vi "Kalman filter_STL.vi"(6 "Previous predicted pixel value":u16, 7 "Kalman gain":fxp<+,16,1>=0.1015625, 8 "Frame number":i32, 9 "Filter gain":fxp<+,16,0>=0.8000030517578125, 10 "Pixel value":u16, 11 "Input valid":bool=TRUE) -> (0 "Kalman filter result":u16, 1 "loop count":i32, 3 "output valid":bool)   [LabVIEW 2015]
uses:
  <vilib>/Platform/TimedLoop/XDataNode/timing_clust.ctl
  <vilib>/Platform/TimedLoop/XDataNode/nitl_modes.ctl
  <vilib>/Platform/TimedLoop/XDataNode/wakeup.ctl
  <vilib>/rvi/Emulation/niFpgaSctlEmulationGetInTimedLoop.vi
  <vilib>/rvi/Emulation/niFpgaEmulationReportErrorSimple.vi
  <vilib>/rvi/Emulation/niFpgaGetClockAttributes.vi
  <vilib>/rvi/Emulation/niFpgaCriticalErrorInLSC.vi
  <vilib>/Platform/TimedLoop/XDataNode/XDataNode.xnode
  <vilib>/rvi/FXPMathLib/FxpSub/XNode/nifxpmath_Sub.xnode
  <vilib>/rvi/FXPMathLib/FxpMul/XNode/nifxpmath_Multiplier.xnode
  <vilib>/rvi/FXPMathLib/FxpAdd/XNode/nifxpmath_Add.xnode
  <vilib>/rvi/FXPMathLib/sim/FxpSim.dll
  <vilib>/Platform/TimedLoop/XDataNode/XDNodeRunTimeDep.lvlib
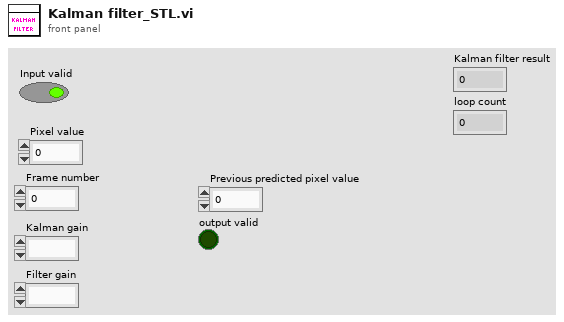
[diagram p1: front panel]
types:
  T1 = typedef "XDNodeRunTimeDep.lvlib/timing_clust.ctl" = cluster{"Expected End [f-1]":u64, "Actual End [f-1]":u64, "Finished Late? [f-1]":bool, "Expected End [i-1]":u64, "Actual End [i-1]":u64, "Finished Late? [i-1]":bool, "Expected Start [i]":u64, "Actual Start [i]":u64, "Expected Start [f]":u64, "Actual Start [f]":u64, "Source Name":string, "Structure Name":string, "Period":i64, "Deadline":i64, "Offset":i64, "Start":i64, "Priority":i32, "Timeout":i32, "Mode":T2, "Wakeup Reason":T3, "Error":errorcluster, "Source Type":string, "Secondary Source Type":string, "Global End Time":u64, "Global Start Time":u64, "Frame Duration":u64, "Iteration Duration":u64, "Assigned CPU":i32, "I/O Scan Engine Mode":u32}
  T2 = typedef "XDNodeRunTimeDep.lvlib/nitl_modes.ctl" = enum32{"No Change", "Process missed periods, maintain original phase", "Discard missed periods, maintain original phase", "Process missed periods, ignore original phase", "Discard missed periods, ignore original phase"}
  T3 = typedef "XDNodeRunTimeDep.lvlib/wakeup.ctl" = enum32{"Normal", "Aborted", "Asynchronous wakeup", "Timing source error", "Timed loop error", "Timeout"}
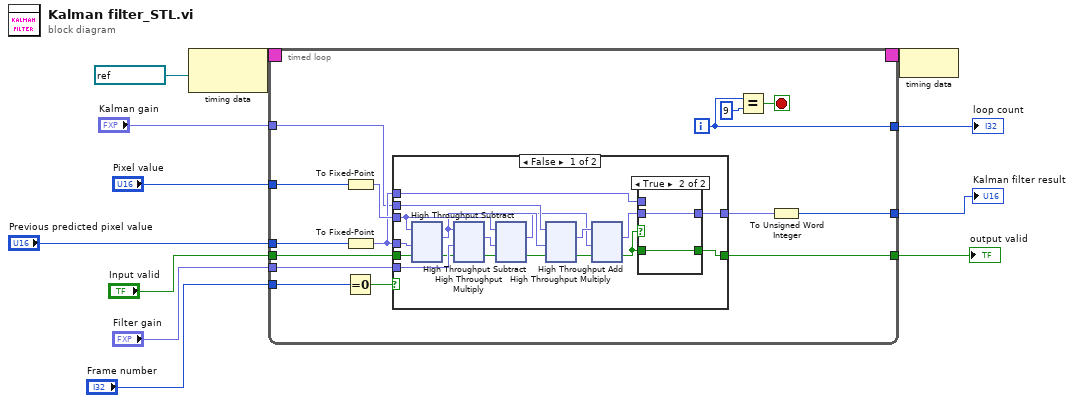
[diagram p0: block diagram]
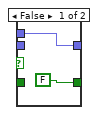
[diagram p2: hidden frame]
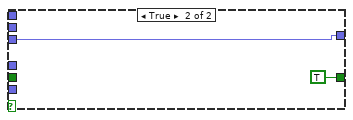
[diagram p3: hidden frame]
diagram:
  n1 = node-c288(refnum<k21> "200MHz" ("Source Name")) -> (w12:T1)
  n2 = timed-loop {
    timing: w12 -> [_]
    timing-out: [_] -> w11
    tunnel: "Frame number" -> [w23]
    tunnel: "Pixel value" -> [w21]
    tunnel: "Kalman gain" -> [w20]
    tunnel: "Filter gain" -> [w18]
    tunnel: [w15] -> w1
    tunnel: "Input valid" -> [w19]
    tunnel: [w24] -> w9
    tunnel: "Previous predicted pixel value" -> [w22]
    tunnel: [w16] -> w2
    i -> [w15]
    stop <- w13 stop-if-true
    n3 = Equal To 0?(x=w23) -> (x = 0?=w27:bool)
    n4 = To Fixed-Point(number=w21) -> (fixed-point=w26:fxp<+,16,16>)  [unwired: 1 in]
    n5 = To Fixed-Point(number=w22) -> (fixed-point=w25:fxp<+,16,16>)  [unwired: 1 in]
    n6 = case shown="False" w27 {
      tunnel: w20 -> [w38 _]
      tunnel: w26 -> [w39 w51]
      tunnel: [w41 w51] -> w17
      tunnel: w25 -> [w45 _]
      tunnel: w19 -> [w33 _]
      tunnel: w18 -> [w36 _]
      tunnel: [w40 TRUE] -> w24
      tunnel: w25 -> [w37 _]
      frame False {
        n7 = xnode "High Throughput Subtract"("x"=w39, "y"=w45, "input valid"=w33) -> ("x-y"=w35:fxp<+/-,18,18>, "output valid"=w32:bool)  [unwired: 1 in, 1 out]
        n8 = xnode ("High Throughput Multiply")("x"=w35, "y"=w36, "input valid"=w32) -> ("x*y"=w44:fxp<+/-,34,18>, "output valid"=w31:bool)  [unwired: 1 in, 1 out]
        n9 = xnode "High Throughput Subtract"("x"=w39, "y"=w44, "input valid"=w31) -> ("x-y"=w34:fxp<+/-,35,19>, "output valid"=w30:bool)  [unwired: 1 in, 1 out]
        n10 = xnode ("High Throughput Multiply")("x"=w38, "y"=w35, "input valid"=w30) -> ("x*y"=w43:fxp<+/-,34,19>, "output valid"=w29:bool)  [unwired: 1 in, 1 out]
        n11 = xnode ("High Throughput Add")("x"=w43, "y"=w34, "input valid"=w29) -> ("x+y"=w42:fxp<+/-,32,20>, "output valid"=w28:bool)  [unwired: 1 in, 1 out]
        n12 = case shown="True" w28 {
          tunnel: w42 -> [_ w49]
          tunnel: w37 -> [w47 _]
          tunnel: [w47 w49] -> w41
          tunnel: [FALSE ("output valid") w48] -> w40
          tunnel: w28 -> [_ w48]
          frame False {
          }
          frame True {
          }
        }
      }
      frame True {
      }
    }
    n13 = Equal?(x=w15, y=9) -> (x = y?=w13:bool)
    n14 = To Unsigned Word Integer(number=w17) -> (unsigned 16bit integer=w16:u16)
  }
  "Kalman filter result" <- w2
  "output valid" <- w9
  "loop count" <- w1
  n15 = node-c288(w11) -> ()
